vi "Convert Configuration to Channels.vi"(8 "error in":errorcluster, 11 "_9216 Config Data":T2={"Conversion Time"=0, "Degree Range"=[], "RTD_Type"=[1], "RTD_A"=[], "RTD_B"=[], "RTD_C"=[], "RTD_Ro"=[]} {"Conversion Time" items=["200 ms", "2.5 ms"]; "Degree Range" items=["Raw Ohms", "Degrees Kelvin", "Degrees Celsius", "Degrees Fahrenheit", "Degrees Rankine"]; "RTD_Type" items=["TCR3851"=1, "TCR3750"=2, "TCR3916"=3, "TCR3920"=4, "TCR3911"=5, "TCR3928"=6, "Custom"=0]}) -> (0 "error out":errorcluster, 2 "Conversion Time":u32(ring) items=["200 ms", "2.5 ms"], 3 "Channels":T1(array[cluster]))   [LabVIEW 2017, in "Modules.lvlib" / "9216.lvclass"]
uses:
  9216.lvclass
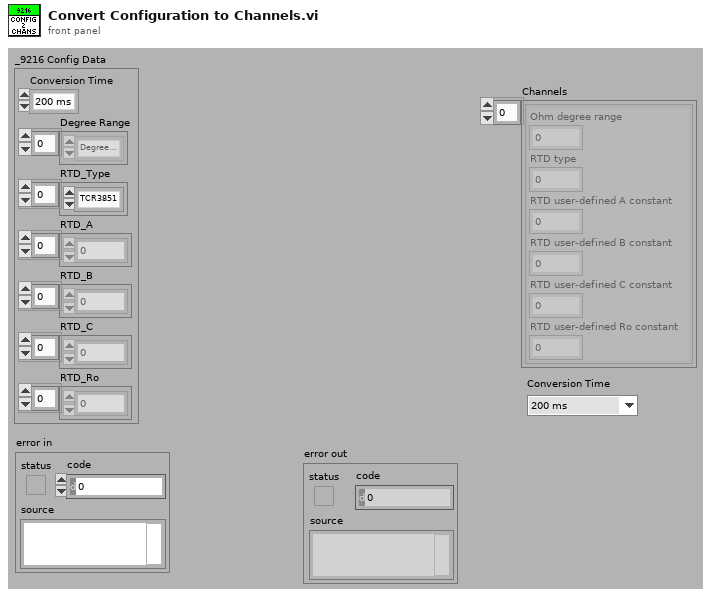
[diagram p1: front panel]
types:
  T1 = cluster{"Ohm degree range":u32, "RTD type":u32, "RTD user-defined A constant":dbl, "RTD user-defined B constant":dbl, "RTD user-defined C constant":dbl, "RTD user-defined Ro constant":dbl}[]
  T2 = cluster{"Conversion Time":u16, "Degree Range":u8[], "RTD_Type":u8[], "RTD_A":dbl[], "RTD_B":dbl[], "RTD_C":dbl[], "RTD_Ro":dbl[]}
  T3 = cluster{"Ohm degree range":u32, "RTD type":u32, "RTD user-defined A constant":dbl, "RTD user-defined B constant":dbl, "RTD user-defined C constant":dbl, "RTD user-defined Ro constant":dbl}
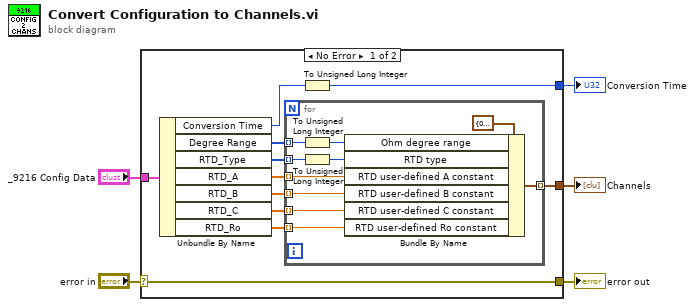
[diagram p0: block diagram]
diagram:
  n1 = case shown="No Error" "error in" {
    selector: "error in" -> [w16 w27]
    tunnel: [w16 w27] -> w4
    tunnel: "_9216 Config Data" -> [w15 _]
    tunnel: [w6 _] -> w2
    tunnel: [w7 _] -> w1
    frame No Error {
      n2 = Unbundle By Name(w15) -> ("Conversion Time"=w13:u16, "Degree Range"=w14:u8[], "RTD_Type"=w12:u8[], "RTD_A"=w11:dbl[], "RTD_B"=w10:dbl[], "RTD_C"=w9:dbl[], "RTD_Ro"=w8:dbl[])
      n3 = for {
        tunnel: w14 -> [w25] mode=indexing
        tunnel: w12 -> [w24] mode=indexing
        tunnel: w11 -> [w23] mode=indexing
        tunnel: w10 -> [w22] mode=indexing
        tunnel: w9 -> [w21] mode=indexing
        tunnel: w8 -> [w20] mode=indexing
        tunnel: [w19] -> w7 mode=indexing
        n4 = To Unsigned Long Integer(number=w25) -> (unsigned 32bit integer=w18:u32)
        n5 = To Unsigned Long Integer(number=w24) -> (unsigned 32bit integer=w17:u32)
        n6 = Bundle By Name(cluster=T3 {"Ohm degree range"=0, "RTD type"=0, "RTD user-defined A constant"=0.0, "RTD user-defined B constant"=0.0, "RTD user-defined C constant"=0.0, "RTD user-defined Ro constant"=0.0} ("Channel"), "Ohm degree range"=w18, "RTD type"=w17, "RTD user-defined A constant"=w23, "RTD user-defined B constant"=w22, "RTD user-defined C constant"=w21, "RTD user-defined Ro constant"=w20) -> (w19:T3)
      }
      n7 = To Unsigned Long Integer(number=w13) -> (unsigned 32bit integer=w6:u32)
    }
    frame Error {
    }
  }
  "Channels" <- w1
  "error out" <- w4
  "Conversion Time" <- w2
